vi "CreateAutoScriptNames.vi"(11 "Index":i32) -> (2 "Concat String":string)   [LabVIEW 2015]
doc: "Create an array"
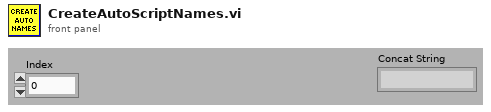
[diagram p1: front panel]
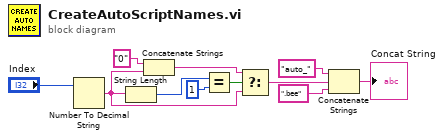
[diagram p0: block diagram]
diagram:
  n1 = Number To Decimal String(number="Index") -> (decimal integer string=w1:string)  [unwired: 1 in]
  n2 = String Length(string=w1) -> (length=w7:i32)
  n3 = Concatenate Strings("0" ("string"), w1) -> (w5:string)
  n4 = Equal?(x=w7, y=1) -> (x = y?=w3:bool)
  n5 = Select(t=w5, s=w3, f=w1) -> (s? t:f=w4:string)
  n6 = Concatenate Strings("auto_" ("string"), w4, ".bee" ("string")) -> (→"Concat String":string)
